vi "XML_EEG_saveFile.vi"(8 "error in (no error)":errorcluster, 10 "XML file path":path, 11 "XML_EEG_File in":refnum<class "XML_EEG_File.lvclass">) -> (0 "error out":errorcluster, 3 "XML_EEG_File out":refnum<class "XML_EEG_File.lvclass">)   [LabVIEW 2016, in "XML_EEG_File_Parser.lvlib" / "XML_EEG_File.lvclass"]
uses:
  XML_EEG_File.lvclass
  XML_EEG_File.lvclass/XML_EEG_File.ctl
  <vilib>/xml/NI_XML.lvlib
panel:
  # "This VI is a part of BCI Design library, http://www.ru-bci.org \nCopyright © 2020, Sotnikov Peter, All rights reserved. License: GNU GPLv3"
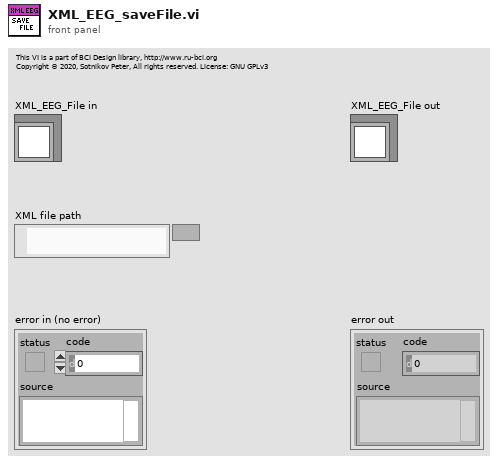
[diagram p1: front panel]
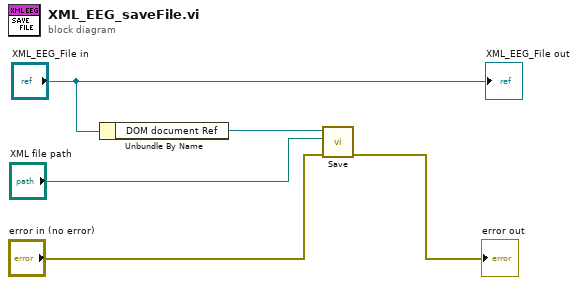
[diagram p0: block diagram]
diagram:
  n1 = Unbundle By Name("XML_EEG_File in") -> ("DOM document Ref"=w5:refnum<k20>)
  n2 = call <vilib>:"Save.vi"("error in (no error)"="error in (no error)", "XML file path"="XML file path", "DOM document in"=w5) -> ("error out"=→"error out":errorcluster)  [unwired: 6 in, 2 out]
  "XML_EEG_File out" <- "XML_EEG_File in"
